vi "菜单选项.vi"(0 "menu reference":refnum<k9>) -> (4 "menu reference out":refnum<k9>, 15 "error out":errorcluster)   [LabVIEW 2014]
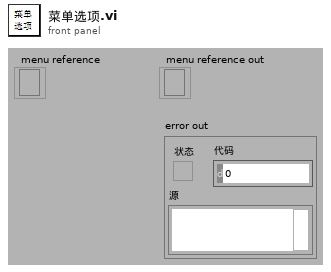
[diagram p1: front panel]
types:
  T1 = cluster{bool, "include Ctrl key?":bool, string}[]
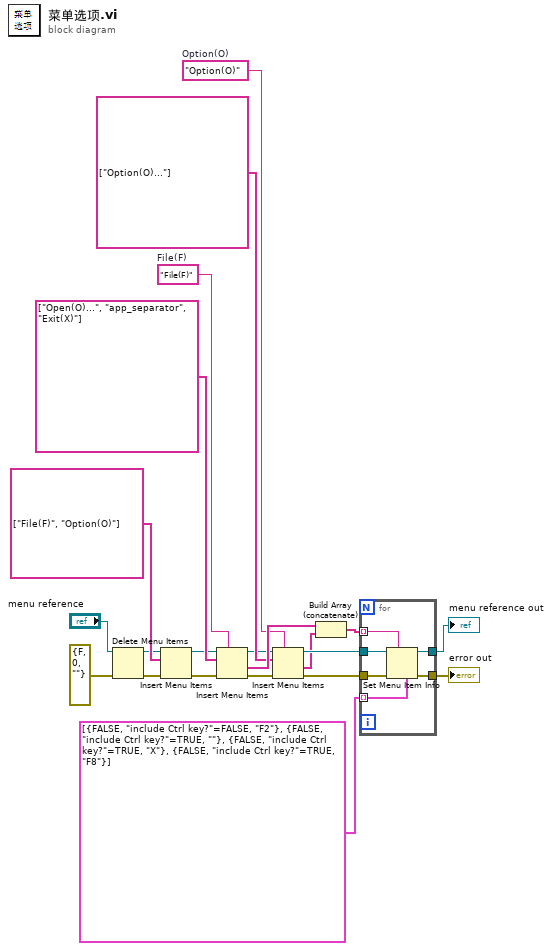
[diagram p0: block diagram]
diagram:
  w8 = "Option(O)"  # Option(O)
  w7 = "File(F)"  # File(F)
  n1 = Delete Menu Items(6:errorcluster {"status"=FALSE, "code"=0, "source"=""} ("错误输入（无错误）"), 9:"menu reference") -> (0:w13:errorcluster, 3:w2:refnum<k9>)  [unwired: 2 in]
  n2 = Insert Menu Items(6:w13, 8:string[] ["File(F)", "Option(O)"] ("项名称"), 9:w2) -> (0:w10:errorcluster, 3:w3:refnum<k9>)  [unwired: 3 in, 1 out]
  n3 = Insert Menu Items(5:w7, 6:w10, 8:string[] ["Open(O)...", "app_separator", "Exit(X)"] ("项名称"), 9:w3) -> (0:w11:errorcluster, 1:w16:string[], 3:w6:refnum<k9>)  [unwired: 2 in]
  n4 = Insert Menu Items(5:w8, 6:w11, 8:string[] ["Option(O)..."] ("项名称"), 9:w6) -> (0:w12:errorcluster, 1:w17:string[], 3:w19:refnum<k9>)  [unwired: 2 in]
  n5 = Build Array (concatenate)(w16, w17) -> (w9:string[])
  n6 = for {
    tunnel: w9 -> [w27] mode=indexing
    tunnel: [w26] -> w20
    tunnel: [w25] -> w21
    tunnel: w12 -> [w24]
    tunnel: T1 [{FALSE, "include Ctrl key?"=FALSE, "F2"}, {FALSE, "include Ctrl key?"=TRUE, ""}, {FALSE, "include Ctrl key?"=TRUE, "X"}, {FALSE, "include Ctrl key?"=TRUE, "F8"}] -> [w23] mode=indexing
    tunnel: w19 -> [w22]
    n7 = Set Menu Item Info(4:w23, 7:w27, 8:w24, 11:w22) -> (0:w25:errorcluster, 3:w26:refnum<k9>)  [unwired: 3 in]
  }
  "error out" <- w21
  "menu reference out" <- w20
